vi "Image_Save_Dequeue.vi"(0 "Data":T2={"Pinch-valve"="Test Sample", "XLP 6000 Pump"="MRJ", "Camera1"="", "Camera2"="", "Img_Capt"=FALSE, "Actuator"=FALSE, "Pump"=FALSE, "Cam 1"=FALSE, "Cam 2"=FALSE, "Empty_Refill"=FALSE, "Crop"=FALSE, "Light intensity"=0, "Exposure Time"=0.0, "Sample Name"="", "Operator"="", "Calibration 1"=path "C:/Users/au540322/Desktop/IHS_Project/images/Debris/Debris_0/Debris_0_2019_06_01-23-32-49-686.PNG", "Calibration 2"=path "C:/Users/au540322/Desktop/IHS_Project/images/Debris/Debris_0/Debris_0_2019_06_01-23-32-49-686.PNG", "Framerate"=1, "Timeout Sample"=1, "Collection date"="", "Sample size threshold"=500, "Empty start"=500, "Command"="", "Station"="", "Species Name"="", "Other Notes"="", "Aperture"=enum."Item 3", "Image Process Queue Size"=100, "Image Save Queue Size"=0, "Overload threshold"=0, "Max Framerate"=0, "Rectangle 1"={"Left"=0, "Top"=0, "Right"=0, "Bottom"=0, "Rotation"=0.0}, "Rectangle 2"={"Left"=0, "Top"=100, "Right"=100, "Bottom"=0, "Rotation"=0.0}, "Detection Region %"=200.0, "Detect 1"=path "C:/Users/au540322/Desktop/IHS_Project/images/Debris/Debris_0/Debris_0_2019_06_01-23-32-49-686.PNG", "Detect 2"=path "C:/Users/au540322/Desktop/IHS_Project/images/Debris/Debris_0/Debris_0_2019_06_01-23-32-49-686.PNG", "Max large object threshold"=500, "Open(T)/Close(F)"=FALSE, "Img_Capt Begin"=FALSE, "Dispense Speed"=0, "Flush Size"=0, "Location"="", "Latitude"="", "Longitude"="", "Determiner"="", "Sex"="", "Camera1_Img"=refnum, "Camera2_Img"=refnum, "Img1_Orig_Disp"=refnum, "Img2_Orig_Disp"=refnum, "Img1_Orig_RGB"=refnum, "Img2_Orig_RGB"=refnum, "Blue_Plane_Extract"=refnum, "Subtracted_Plane"=refnum, "Img1_Binary"=refnum, "Img2_Binary"=refnum, "Crop_Mask"=refnum, "Img1_Save"=refnum, "Img2_Save"=refnum, "Img1_Cali_Full"=refnum, "Img2_Cali_Full"=refnum, "Img1_Cali_Detect"=refnum, "Img2_Cali_Detect"=refnum, "Cam 1 queue"=refnum, "Cam 2 queue"=refnum, "Cam 1 - save queue"=refnum, "Cam 2 - save queue"=refnum, "Overlay_Ring"=0, "SystemVersion"=0, "System Serial"="", "Legacy Cam Attributes"=FALSE, "Camera Orientation 1"="", "Camera Orientation 2"="", "Pixel to mm 1"=0.0, "Pixel to mm 2"=0.0, "CAM1 Model"=enum."a2A5328-15ucBAS", "CAM2 Model"=enum."a2A5328-15ucBAS", "Flush Insect"=FALSE, "Pump Size"=FALSE, "Barcode"="", "Phase3"=FALSE, "Mega F3"="", "Container nr."=0.0, "Flush Error"=TRUE, "Start System"=FALSE, "Size Interval"=0.0, "Mun. of containers"=0.0, "Sorting sys."=FALSE, "Initial size"=0.0} {"SystemVersion" items=["Standard", "XL"]; "Overlay_Ring" items=["Session Data", "Extended Setup", "Buffer", "Camera", "Dispenser", "Stats", "Connections"]; "Flush Size" min=1; "Dispense Speed" min=1; "Rectangle 2"."Rotation" format="%.2f"; "Rectangle 2"."Left" scale=0.0..1024.0; "Rectangle 2"."Right" scale=0.0..1024.0; "Rectangle 1"."Rotation" format="%.2f"; "Rectangle 1"."Left" scale=0.0..1024.0; "Rectangle 1"."Right" scale=0.0..1024.0; "Max Framerate" min=1; "Overload threshold" min=1; "Image Save Queue Size" min=1; "Image Process Queue Size" min=1; "Empty start" min=1; "Sample size threshold" min=1; "Framerate" min=1; "Light intensity" scale=0.0..100.0}, 2 "Camera":T5, 3 "Old":i32, 4 "cam1_prev":u32, 5 "Other":i32, 6 "Queue active":bool, 7 "cam2_prev":u32) -> (16 "timed out?":bool, 17 "Sample Data":dbl[](array[numeric]), 20 "# elements in queue":i32, 22 "State out":i32, 23 "Image Save 1":T1, 24 "cam1_count":u32, 25 "Image Save 2":T1, 26 "Last image":bool, 27 "cam2_count":u32)   [LabVIEW 2024]
uses:
  Camera_ID.ctl
  controls/Data.ctl
  <vilib>/userDefined/High Color/IMAQdx.ctl
  <vilib>/vision/Image Controls.llb/IMAQ Image.ctl
panel:
  out "error out 3":errorcluster
  out "error out 2":errorcluster
  out "error out":errorcluster
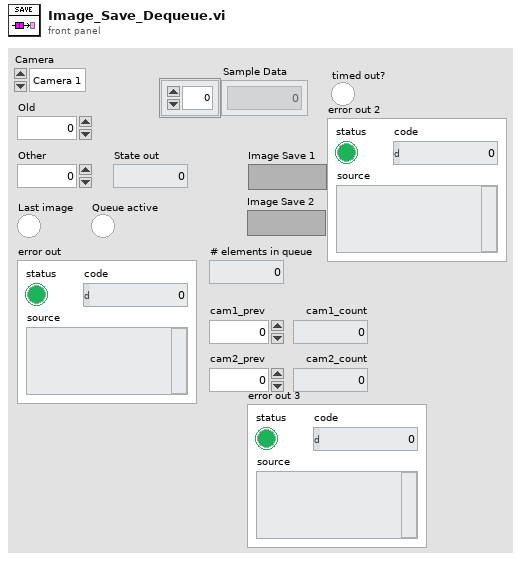
[diagram p1: front panel]
types:
  T1 = typedef "IMAQ Image.ctl" = refnum<image>
  T2 = typedef "Data.ctl" = cluster{"Pinch-valve":refnum<visa-resource-name>, "XLP 6000 Pump":refnum<visa-resource-name>, "Camera1":T3, "Camera2":T3, "Img_Capt":bool, "Actuator":bool, "Pump":bool, "Cam 1":bool, "Cam 2":bool, "Empty_Refill":bool, "Crop":bool, "Light intensity":i32, "Exposure Time":dbl, "Sample Name":string, "Operator":string, "Calibration 1":path, "Calibration 2":path, "Framerate":i32, "Timeout Sample":i32, "Collection date":string, "Sample size threshold":i32, "Empty start":u32, "Command":string, "Station":string, "Species Name":string, "Other Notes":string, "Aperture":enum32{"Item 0", "Item 1", "Item 2", "Item 3"}, "Image Process Queue Size":i32, "Image Save Queue Size":i32, "Overload threshold":i32, "Max Framerate":i32, "Rectangle 1":T4, "Rectangle 2":T4, "Detection Region %":dbl, "Detect 1":path, "Detect 2":path, "Max large object threshold":i32, "Open(T)/Close(F)":bool, "Img_Capt Begin":bool, "Dispense Speed":i32, "Flush Size":i32, "Location":string, "Latitude":string, "Longitude":string, "Determiner":string, "Sex":string, "Camera1_Img":T1, "Camera2_Img":T1, "Img1_Orig_Disp":T1, "Img2_Orig_Disp":T1, "Img1_Orig_RGB":T1, "Img2_Orig_RGB":T1, "Blue_Plane_Extract":T1, "Subtracted_Plane":T1, "Img1_Binary":T1, "Img2_Binary":T1, "Crop_Mask":T1, "Img1_Save":T1, "Img2_Save":T1, "Img1_Cali_Full":T1, "Img2_Cali_Full":T1, "Img1_Cali_Detect":T1, "Img2_Cali_Detect":T1, "Cam 1 queue":refnum<queue>, "Cam 2 queue":refnum<queue>, "Cam 1 - save queue":refnum<queue>, "Cam 2 - save queue":refnum<queue>, "Overlay_Ring":u16, "SystemVersion":u16, "System Serial":string, "Legacy Cam Attributes":bool, "Camera Orientation 1":string, "Camera Orientation 2":string, "Pixel to mm 1":dbl, "Pixel to mm 2":dbl, "CAM1 Model":enum16{"a2A5328-15ucBAS", "acA1920-155uc"}, "CAM2 Model":enum16{"a2A5328-15ucBAS", "acA1920-155uc"}, "Flush Insect":bool, "Pump Size":bool, "Barcode":string, "Phase3":bool, "Mega F3":refnum<visa-resource-name>, "Container nr.":dbl, "Flush Error":bool, "Start System":bool, "Size Interval":dbl, "Mun. of containers":dbl, "Sorting sys.":bool, "Initial size":dbl}
  T3 = typedef "IMAQdx.ctl" = refnum<k21>
  T4 = typedef "IMAQ Rectangle" = cluster{"Left":i32, "Top":i32, "Right":i32, "Bottom":i32, "Rotation":dbl}
  T5 = typedef "Camera_ID.ctl" = enum16{"Camera 1", "Camera 2"}
  T6 = cluster{"Timestamp":string, "Image Pixels (U32)":u32[][], "Prev. sample":i32, "Sample Data":dbl[], "output cluster":cluster{"Global Rectangle":i32[], "Contours":cluster{"ID":enum32{"External", "Internal"}, "Type":u32, "Coordinates":i32[]}[]}}
  T7 = cluster{"Global Rectangle":i32[], "Contours":cluster{"ID":enum32{"External", "Internal"}, "Type":u32, "Coordinates":i32[]}[]}
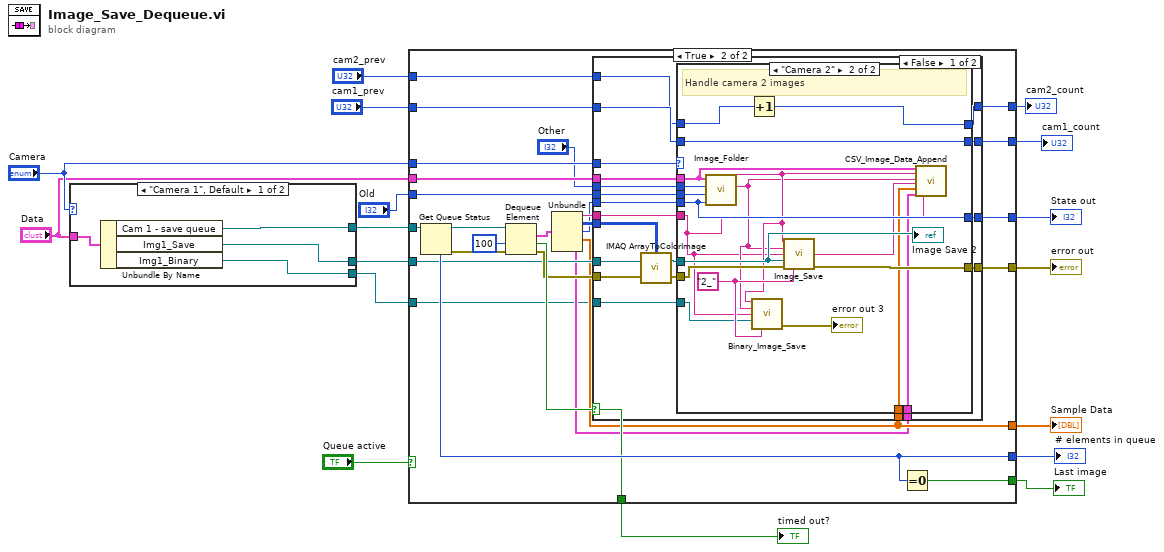
[diagram p0: block diagram]
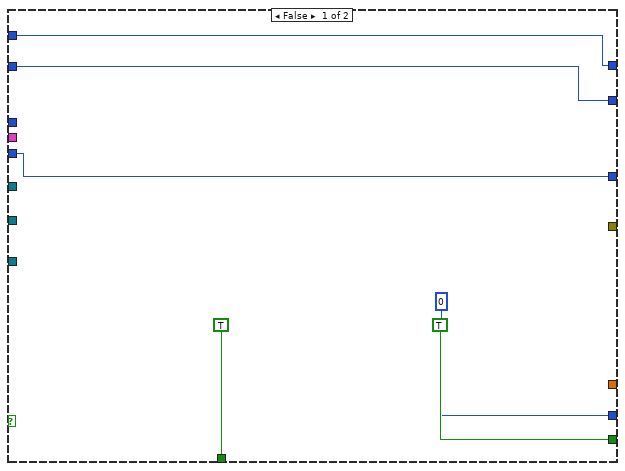
[diagram p2: hidden frame]
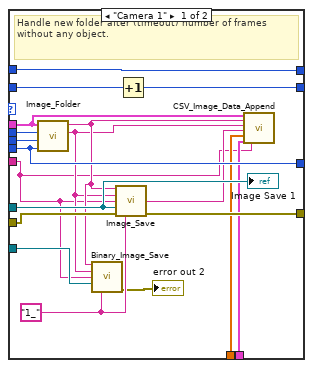
[diagram p3: hidden frame]
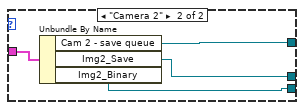
[diagram p5: hidden frame]
diagram:
  n1 = case shown="\"Camera 1\", Default" "Camera" {
    tunnel: [w20 w25] -> w16
    tunnel: "Data" -> [w21 w24]
    tunnel: [w19 w23] -> w6
    tunnel: [w18 w22] -> w1
    frame "Camera 1", Default {
      n2 = Unbundle By Name(w21) -> ("Cam 1 - save queue"=w20:refnum<queue>, "Img1_Save"=w19:T1, "Img1_Binary"=w18:T1)
    }
    frame "Camera 2" {
      n3 = Unbundle By Name(w24) -> ("Cam 2 - save queue"=w25:refnum<queue>, "Img2_Save"=w23:T1, "Img2_Binary"=w22:T1)
    }
  }
  n4 = case shown="True" "Queue active" {
    tunnel: "Camera" -> [_ w57]
    tunnel: w16 -> [_ w53]
    tunnel: "Data" -> [_ w52]
    tunnel: [0 ("# elements in queue") w51] -> w13
    tunnel: [TRUE w50] -> w12
    tunnel: [_ w49] -> w11
    tunnel: [w29 w44] -> w10
    tunnel: "Old" -> [w29 w43]
    tunnel: [_ w38] -> w8
    tunnel: [TRUE ("timed out?") w41] -> w7
    tunnel: w6 -> [_ w39]
    tunnel: [w27 w36] -> w5
    tunnel: "cam1_prev" -> [w27 w35]
    tunnel: "cam2_prev" -> [w26 w34]
    tunnel: [w26 w33] -> w2
    tunnel: w1 -> [_ w32]
    frame False {
    }
    frame True {
      n5 = Get Queue Status(queue=w53) -> (queue out=w54:refnum<queue>, error out=w47:errorcluster, # elements in queue=w51:i32)  [unwired: 2 in, 5 out]
      n6 = Dequeue Element(queue=w54, timeout in ms (-1)=100, error in (no error)=w47) -> (element=w56:T6, timed out?=w41:bool, error out=w40:errorcluster)  [unwired: 1 out]
      n7 = Unbundle(w56) -> ("Timestamp"=w48:string, "Image Pixels (U32)"=w55:u32[][], "Prev. sample"=w46:i32, "Sample Data"=w38:dbl[], "output cluster"=w37:T7)
      n8 = case shown="False" w41 {
        tunnel: w57 -> [w77 _]
        tunnel: w55 -> [w65 _]
        tunnel: w52 -> [w76 _]
        tunnel: [w75 w118] -> w49
        tunnel: w48 -> [w74 _]
        tunnel: w46 -> [w73 _]
        tunnel: "Other" -> [w72 _]
        tunnel: [w71 w119] -> w44
        tunnel: w43 -> [w70 w119]
        tunnel: w40 -> [w66 w118]
        tunnel: w39 -> [w69 _]
        tunnel: w38 -> [w64 _]
        tunnel: w37 -> [w63 _]
        tunnel: [w62 w117] -> w36
        tunnel: w35 -> [w61 w117]
        tunnel: w34 -> [w60 w116]
        tunnel: [w59 w116] -> w33
        tunnel: w32 -> [w58 _]
        frame False {
          n9 = call "IMAQ ArrayToColorImage"("Image Pixels (U32)"=w65, "Image"=w69, "error in (no error)"=w66) -> ("Image Out"=w68:T1, "error out"=w67:errorcluster)  [unwired: 2 in]
          n10 = case shown="\"Camera 2\"" w77 {
            tunnel: [w96 w115] -> w75
            tunnel: w68 -> [w91 w110]
            tunnel: w76 -> [w90 w109]
            tunnel: w74 -> [w79 w98]
            tunnel: w67 -> [w95 w114]
            tunnel: w73 -> [w92 w111]
            tunnel: w70 -> [w94 w113]
            tunnel: w72 -> [w93 w112]
            tunnel: [w92 w111] -> w71
            tunnel: w64 -> [w88 w107]
            tunnel: w63 -> [w87 w106]
            tunnel: [w86 w103] -> w62
            tunnel: w61 -> [w85 w103]
            tunnel: w60 -> [w84 w105]
            tunnel: [w84 w104] -> w59
            tunnel: w58 -> [w83 w99]
            frame "Camera 1" {
              w80 = "1_" ("Camera image prefix")
              # "Handle new folder after (timeout) number of frames without any object."
              n11 = call "Image_Folder.vi"("New"=w92, "Old"=w94, "Other"=w93, "input cluster"=w90) -> ("Subfolder Name"=w81:string, "Subfolder Path"=w82:string)  [unwired: 6 in]
              n12 = call "Binary_Image_Save.vi"("Subfolder path"=w82, "Subfolder Name"=w81, "Timestamp"=w79, "Image in"=w83, "Camera"=w80) -> ("error out"=→"error out 2":errorcluster)  [unwired: 7 in, 3 out]
              n13 = call "Image_Save.vi"("Subfolder path"=w82, "Subfolder Name"=w81, "Timestamp"=w79, "Image in"=w91, "error in"=w95, "Camera"=w80) -> ("Image Name"=w89:string, "error out"=w96:errorcluster)  [unwired: 6 in, 2 out]
              n14 = Increment(x=w85) -> (x+1=w86:u32)
              n15 = call "CSV_Image_Data_Append.vi"("input cluster"=w90, "Image path"=w82, "Sample Name"=w81, "Image Name"=w89, "Sample Data"=w88, "ROI Descriptor"=w87, "Timestamp"=w79) -> ()  [unwired: 13 in]
              "Image Save 1" <- w91
            }
            frame "Camera 2" {
              w102 = "2_" ("Camera image prefix")
              # "Handle camera 2 images"
              n16 = call "Image_Folder.vi"("New"=w111, "Old"=w113, "Other"=w112, "input cluster"=w109) -> ("Subfolder Name"=w100:string, "Subfolder Path"=w101:string)  [unwired: 6 in]
              n17 = Increment(x=w105) -> (x+1=w104:u32)
              n18 = call "Binary_Image_Save.vi"("Subfolder path"=w101, "Subfolder Name"=w100, "Timestamp"=w98, "Image in"=w99, "Camera"=w102) -> ("error out"=→"error out 3":errorcluster)  [unwired: 7 in, 3 out]
              n19 = call "Image_Save.vi"("Subfolder path"=w101, "Subfolder Name"=w100, "Timestamp"=w98, "Image in"=w110, "error in"=w114, "Camera"=w102) -> ("Image Name"=w108:string, "error out"=w115:errorcluster)  [unwired: 6 in, 2 out]
              n20 = call "CSV_Image_Data_Append.vi"("input cluster"=w109, "Image path"=w101, "Sample Name"=w100, "Image Name"=w108, "Sample Data"=w107, "ROI Descriptor"=w106, "Timestamp"=w98) -> ()  [unwired: 13 in]
              "Image Save 2" <- w110
            }
          }
        }
        frame True {
        }
      }
      n21 = Equal To 0?(x=w51) -> (x = 0?=w50:bool)
    }
  }
  "# elements in queue" <- w13
  "Last image" <- w12
  "error out" <- w11
  "State out" <- w10
  "Sample Data" <- w8
  "timed out?" <- w7
  "cam1_count" <- w5
  "cam2_count" <- w2
